vi "Make_file_path.vi"(10 "File Name String":string="Test", 11 "Base path":path=path "C:/Users/MPI/Documents/Test Saving Data") -> (4 "TDMS path":path=path "C:/Users/MPI/Documents/MPS Operation/MATLAB/DataTemp/Jan_2022_06/2022_01_06_23_02_44_Test.tdms")   [LabVIEW 2022 SP3]
panel:
  out "Total File Name":string="Jan_2022_06\\2022_01_06_23_02_44_Test.tdms"
  # "Used when storing in HDF format"
  # "Used when storing time domain"
  # "Used when storing in TDMS format"
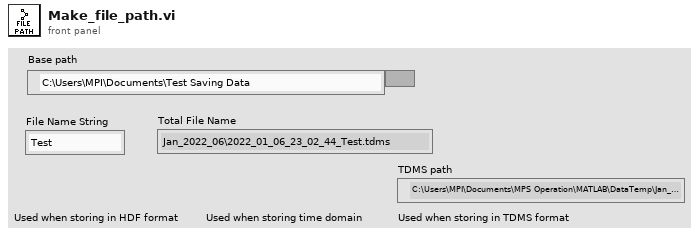
[diagram p1: front panel]
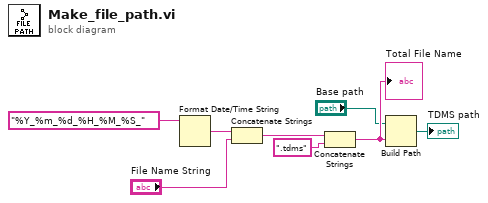
[diagram p0: block diagram]
diagram:
  n1 = Format Date/Time String(time format string (%c)="%Y_%m_%d_%H_%M_%S_") -> (date/time string=w1:string)  [unwired: 2 in]
  n2 = Concatenate Strings(w1, "File Name String") -> (w3:string)
  n3 = Concatenate Strings(w3, ".tdms" ("string")) -> (w5:string)
  "Total File Name" <- w5
  n4 = Build Path(base path="Base path", name or relative path=w5) -> (appended path=→"TDMS path":path)
